vi "Transfer Immediate Wrapper.vi"() -> ()   [LabVIEW 2019]
panel:
  in  "Synchronication":enum16{"Start", "Wait"}(ring)
  in  "Duration":dbl
  in  "Setpoint":dbl
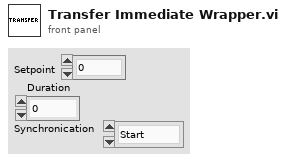
[diagram p1: front panel]
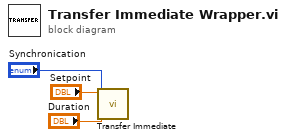
[diagram p0: block diagram]
diagram:
  n1 = call "Transfer Immediate.vi"("Synchronication"="Synchronication", "Duration"="Duration", "Setpoint"="Setpoint") -> ()  [unwired: 8 in, 1 out]
